vi "TVEMePe_2.vi"(8 "error in (no error)":errorcluster, 10 "Fluke":dbl[][](array[numeric]), 11 "NIST":dbl[][](array[numeric])) -> (0 "error out":errorcluster, 3 "TVEMePe":dbl[][](array[numeric]))   [LabVIEW 2014]
uses:
  <vilib>/Analysis/coordinate.llb/Angle Units.ctl
  <vilib>/Analysis/coordinate.llb/Angle Range (Degree).ctl
  <vilib>/Analysis/coordinate.llb/Wrap Angle (scalar).vi
  <vilib>/Analysis/NI_AAL_Angle.lvlib
panel:
  out "Waveform Chart":dbl[][](graph)
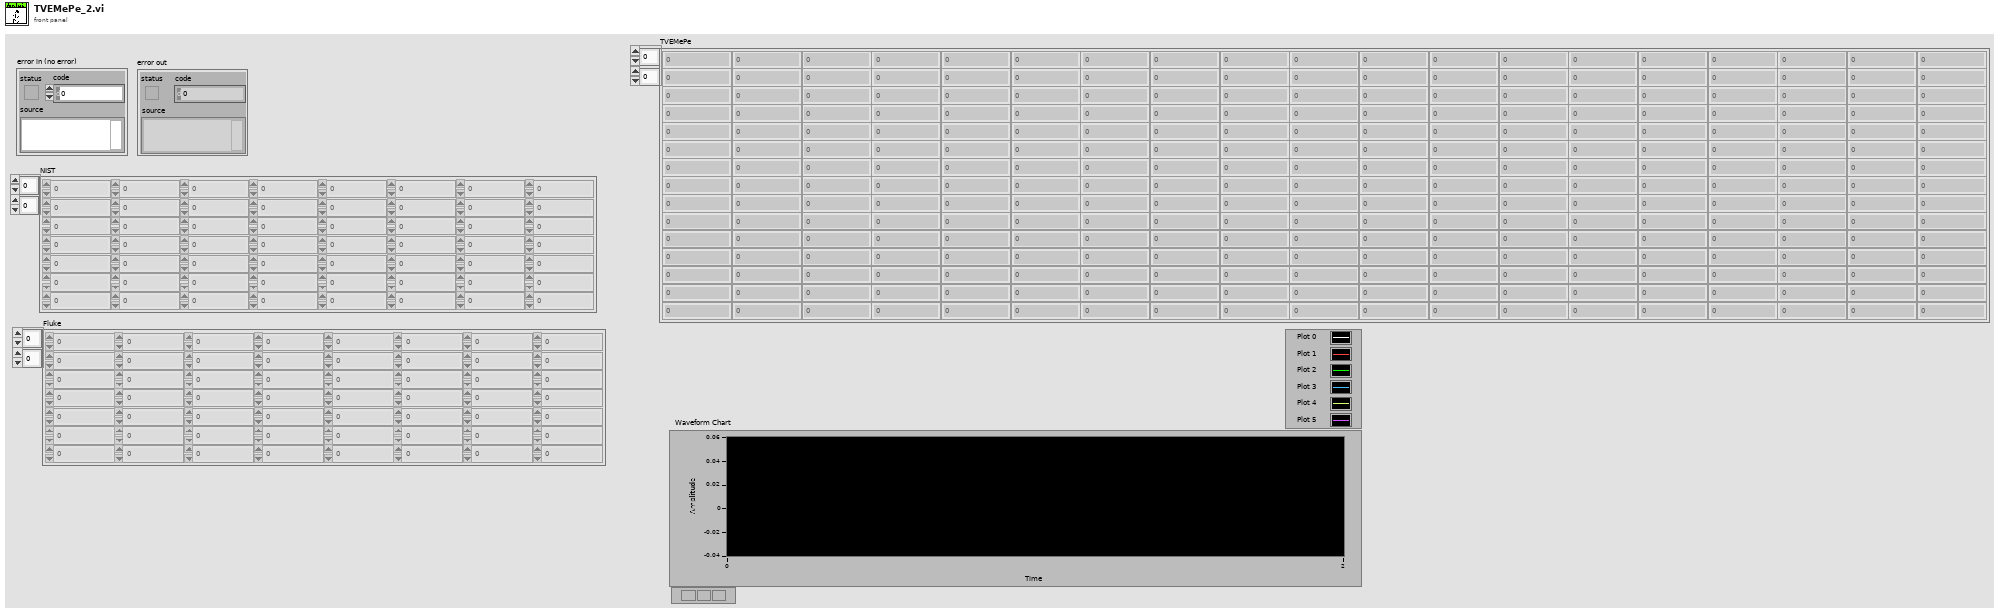
[diagram p1: front panel]
types:
  T1 = typedef "NI_AAL_Angle.lvlib/Angle Range (Degree).ctl" = u16
  T2 = typedef "NI_AAL_Angle.lvlib/Angle Units.ctl" = i32
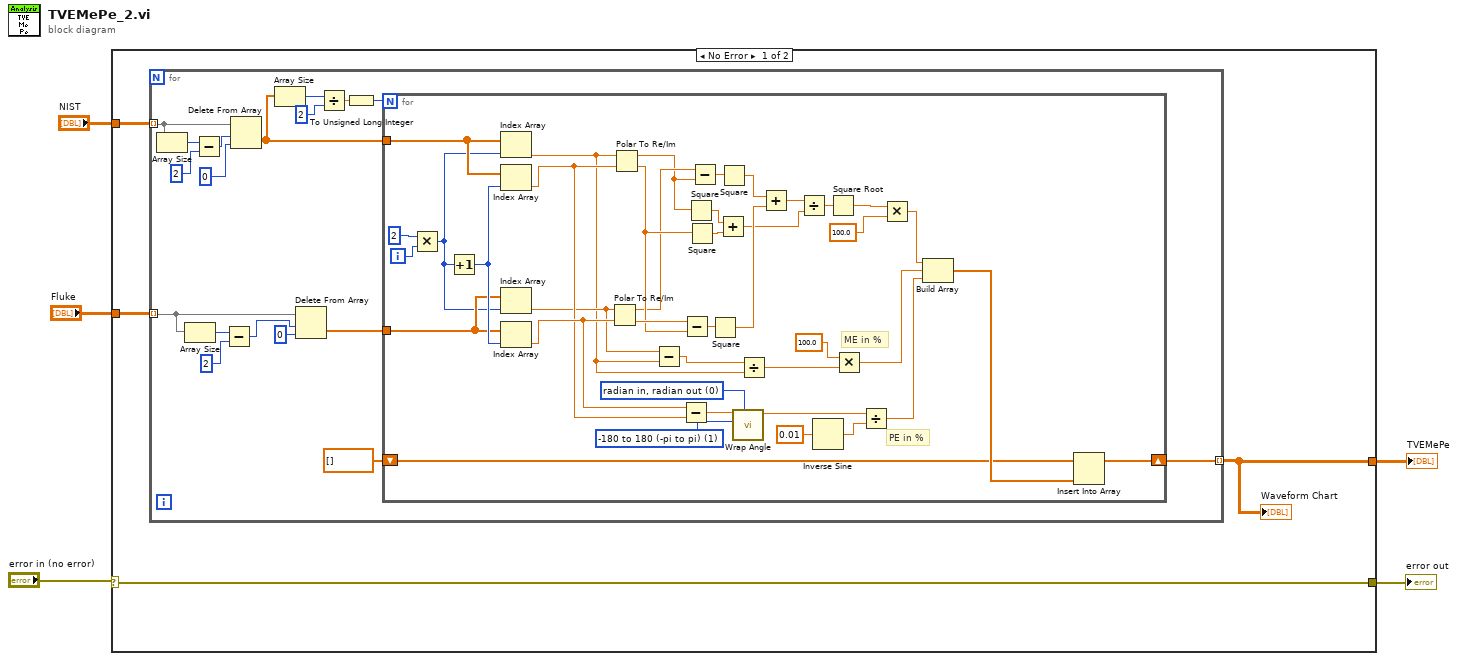
[diagram p0: block diagram]
diagram:
  n1 = case shown="No Error" "error in (no error)" {
    selector: "error in (no error)" -> [w9 w69]
    tunnel: [w9 w69] -> w4
    tunnel: "Fluke" -> [w8 _]
    tunnel: "NIST" -> [w7 _]
    tunnel: [w6 dbl[][] []] -> w3
    frame No Error {
      n2 = for {
        tunnel: w8 -> [w13] mode=indexing
        tunnel: w7 -> [w12] mode=indexing
        tunnel: [w10] -> w6 mode=indexing
        n3 = Array Size(array=w12) -> (size(s)=w25:i32)
        n4 = Array Size(array=w13) -> (size(s)=w22:i32)
        n5 = Subtract(x=w25, y=2) -> (x-y=w27:i32)
        n6 = Subtract(x=w22, y=2) -> (x-y=w20:i32)
        n7 = Delete From Array(array=w12, length=w27, index=0) -> (deleted portion=w18:dbl[])  [unwired: 1 out]
        n8 = Array Size(array=w18) -> (size(s)=w17:i32)
        n9 = Delete From Array(array=w13, length=w20, index=0) -> (deleted portion=w19:dbl[])  [unwired: 1 out]
        n10 = Divide(x=w17, y=2) -> (x/y=w15:dbl)
        n11 = To Unsigned Long Integer(number=w15) -> (unsigned 32bit integer=w14:u32)
        n12 = for {
          N: w14 -> [_]
          tunnel: w19 -> [w64]
          tunnel: w18 -> [w63]
          shift-right: [w41] -> w10
          shift-left: dbl[] [] -> [w39]
          i -> [w67]
          w44 = T1 1 items=["none", "-180 to 180 (-pi to pi)", "0 to 360 (0 to 2pi)"] ("angle range")
          w45 = T2 0 items=["radian in, radian out", "radian in, degree out", "degree in, degree out", "degree in, radian out"] ("angle units")
          # "PE in %"
          # "ME in %"
          n13 = Multiply(x=2, y=w67) -> (x*y=w48:i32)
          n14 = Increment(x=w48) -> (x+1=w65:i32)
          n15 = Index Array(array=w63, index=w48) -> (element=w34:dbl)
          n16 = Index Array(array=w63, index=w65) -> (element=w46:dbl)
          n17 = Index Array(array=w64, index=w48) -> (element=w35:dbl)
          n18 = Index Array(array=w64, index=w65) -> (element=w47:dbl)
          n19 = Polar To Re/Im(2:w47, 3:w35) -> (0:w51:dbl, 1:w49:dbl)
          n20 = Polar To Re/Im(2:w46, 3:w34) -> (0:w50:dbl, 1:w28:dbl)
          n21 = Subtract(x=w35, y=w34) -> (x-y=w33:dbl)
          n22 = Subtract(x=w47, y=w46) -> (x-y=w43:dbl)
          n23 = Subtract(x=w51, y=w50) -> (x-y=w61:dbl)
          n24 = Square(x=w28) -> (x^2=w58:dbl)
          n25 = Square(x=w50) -> (x^2=w57:dbl)
          n26 = Subtract(x=w49, y=w28) -> (x-y=w62:dbl)
          n27 = Square(x=w61) -> (x^2=w59:dbl)
          n28 = Add(x=w58, y=w57) -> (x+y=w55:dbl)
          n29 = Square(x=w62) -> (x^2=w60:dbl)
          n30 = call-poly <vilib>:"Wrap Angle.vi"("angle units"=w45, "angle range"=w44, "angle in"=w43) -> ("angle out"=w30:dbl)  [unwired: 7 in, 1 out]
          n31 = Divide(x=w33, y=w34) -> (x/y=w36:dbl)
          n32 = Add(x=w60, y=w59) -> (x+y=w56:dbl)
          n33 = Divide(x=w56, y=w55) -> (x/y=w54:dbl)
          n34 = Inverse Sine(1:0.01 ("x")) -> (0:w31:dbl)
          n35 = Square Root(x=w54) -> (sqrt(x)=w53:dbl)
          n36 = Multiply(x=100.0, y=w36) -> (x*y=w37:dbl)
          n37 = Divide(x=w30, y=w31) -> (x/y=w29:dbl)
          n38 = Multiply(x=w53, y=100.0 ("sqrt(x)")) -> (x*y=w42:dbl)
          n39 = Build Array(w42, w37, w29) -> (w40:dbl[])
          n40 = Insert Into Array(array=w39, new element=w40) -> (w41:dbl[])  [unwired: 1 in]
        }
      }
      "Waveform Chart" <- w6
    }
    frame Error {
    }
  }
  "error out" <- w4
  "TVEMePe" <- w3
